vi "CTRE_PigeonIMU_UpdateUsage.vi"(10 "Usage":T1 items=["Defaul"=0, "ConnectCAN"=1, "ConnectTalonSRX"=2, "GetCompass"=134217728, "GetYPR"=268435456, "GetFused"=536870912, "GetAccel"=1073741824, "TempComp"=2147483648], 11 "PigeonIMUDevRef":T2={"DeviceStatus"={"status"=FALSE, "code"=0, "source"=""}, "Device Number"=0, "Type"=352321536, "Device ID"=0} {"Type" items=["CAN"=352321536, "TalonSRX"=33554432]}) -> ()   [LabVIEW 2016]
uses:
  <vilib>/Rock Robotics/WPI/ThirdParty/Sensors/Pigeon IMU/CTRE_PigeonIMU_DeviceRef.ctl
  <vilib>/Rock Robotics/WPI/ThirdParty/Sensors/Pigeon IMU/CTRE_PigeonIMU_ConnectionType.ctl
  <vilib>/Rock Robotics/WPI/ThirdParty/Sensors/Pigeon IMU/CTRE_PigeonIMU_UsageTypes.ctl
  <vilib>/Rock Robotics/WPI/ThirdParty/Sensors/Pigeon IMU/CTRE_PigeonIMU_GlobalOps.ctl
  <vilib>/Rock Robotics/WPI/ThirdParty/CanMotor/TalonSRX/WPI_CANTalonSRX_GlobalOps.ctl
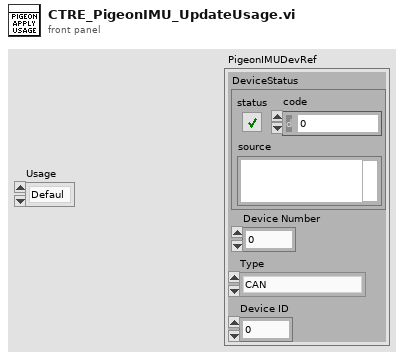
[diagram p1: front panel]
types:
  T1 = typedef "CTRE_PigeonIMU_UsageTypes.ctl" = u32
  T2 = typedef "CTRE_PigeonIMU_DeviceRef.ctl" = cluster{"DeviceStatus":errorcluster, "Device Number":u8, "Type":T3, "Device ID":u32}
  T3 = typedef "CTRE_PigeonIMU_ConnectionType.ctl" = u32
  T4 = typedef "CTRE_PigeonIMU_GlobalOps.ctl" = enum16{"Read For Send", "Write Error", "Get All", "Set Control Frame Rate", "Set Enable Frame Rate", "Write After Receive Fused Heading", "Write After Receive YPR", "Write After Receive Status", "Write After Receive Raw Magnetomoter", "Write After Receive Biased Magnetometer", "Write After Receive Biased Accelerometer", "Write After Receive Gyro", "Write After Receive Acceleromter Angles", "Write After Receive Startup Status", "Write After Receive Compass", "Write After Receive Quaternian", "Write After Receive AccumGyro", "Set Usage Frame"}
  T5 = typedef "CTRE_PigeonIMU_GlobalStatus.ctl" = cluster{"PigeonState":T6, "FusedHeading":cluster{"Heading":dbl, "Valid?":bool, "Fusing?":bool}, "YPR":cluster{"Yaw":dbl, "Pitch":dbl, "Roll":dbl}, "Compass":cluster{"Heading":dbl, "Magnitude":dbl, "Absolute Heading":dbl}, "Accelerometer":cluster{"Biased":cluster{"X":i16, "Y":i16, "Z":i16, "Norm":i16}, "Angles":cluster{"XZ Tilt":dbl, "YZ Tilt":dbl, "XY Tilt":dbl}}, "Magnetometer":cluster{"Raw":cluster{"X":i16, "Y":i16, "Z":i16}, "Biased":cluster{"X":i16, "Y":i16, "Z":i16}}, "Gyro":cluster{"X":dbl, "Y":dbl, "Z":dbl, "Norm":dbl}, "6D Quaternian":cluster{"W":dbl, "X":dbl, "Y":dbl, "Z":dbl}, "Temp. (C)":dbl, "UpTime":u32, "StartupStatus":cluster{"ResetCount":i32, "ResetFlags":i32, "FirmwareVersion":i32, "HasReset?":bool}, "Calibration":cluster{"CurrentMode":T7, "LastCalError":i32, "CalBooting?":bool}, "CAN Error":errorcluster, "AccumGyro":cluster{"X":dbl, "Y":dbl, "Z":dbl}, "Usage Frame":u32}
  T6 = typedef "CTRE_PigeonIMU_PigeonState.ctl" = enum16{"NoComm", "Initializing", "Ready", "UserCalibration"}
  T7 = typedef "CTRE_PigeonIMU_CalibrationMode.ctl" = u16
  T8 = typedef "WPI_CANTalonSRX_GlobalOps.ctl" = enum16{"Read For Send", "Write After Receive General", "Write After Receive Feedback", "Write After Receive Encoder", "Write After Receive Ain", "Write Error", "Get All", "Set Output", "Set Mode", "Set Master ID", "Set Brake Mode", "Set Reverse Feedback Sensor", "Set Reverse Closed Loop Output", "Set Override Limits", "Set Forward Limit Enabled", "Set Reverse Limit Enabled", "Set Feedback Select", "Set Profile Select", "Set Throttle Ramp Rate", "Disable", "Set Enc Codes Per Rev", "Set Num Pot Turns", "Set Control Frame Rate", "Enable Legacy Control", "Write After Receive Pulse Width", "Set Enable Frame Rate", "Write After Receive Motion Profile", "Set Motion Profile Flow Control", "Set Motion Profile Control Frame Rate", "Set Current Limit Enable", "Set Usage Frame"}
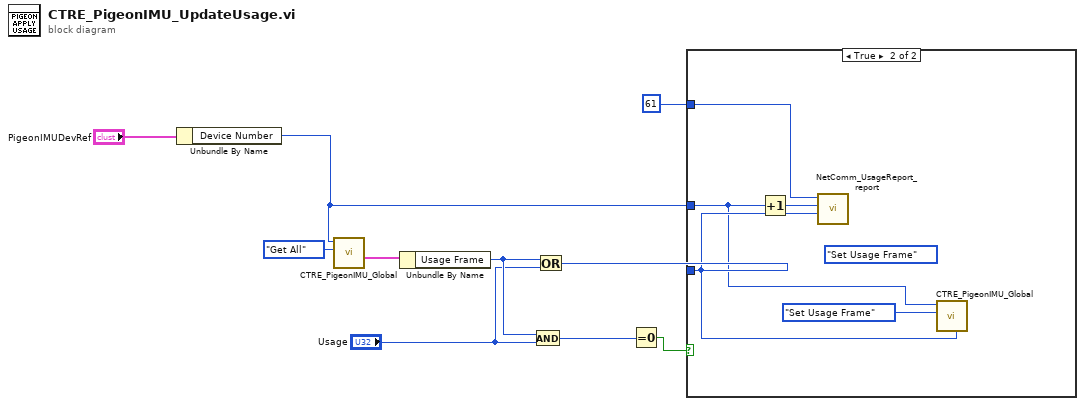
[diagram p0: block diagram]
diagram:
  n1 = Unbundle By Name("PigeonIMUDevRef") -> ("Device Number"=w2:u8)
  n2 = call <vilib>:"CTRE_PigeonIMU_Global.vi"("Operation"=CTRE_PigeonIMU_GlobalOps."Get All", "Device ID (0)"=w2) -> ("Get All"=w4:T5)  [unwired: 7 in, 2 out]
  n3 = Unbundle By Name(w4) -> ("Usage Frame"=w3:u32)
  n4 = And(x=w3, y="Usage") -> (x .and. y?=w9:T1)
  n5 = Or(x=w3, y="Usage") -> (x .or. y?=w8:T1)
  n6 = Equal To 0?(x=w9) -> (x = 0?=w10:bool)
  n7 = case shown="True" w10 {
    tunnel: 61 -> [_ w15]
    tunnel: w2 -> [_ w11]
    tunnel: w8 -> [_ w12]
    frame False {
    }
    frame True {
      (unwired) WPI_CANTalonSRX_GlobalOps."Set Usage Frame" ("Operation")
      n8 = Increment(x=w11) -> (x+1=w14:u8)
      n9 = call <vilib>:"NetComm_UsageReport_report.vi"("Context"=w12, "Instance Number"=w14, "Resource Type"=w15) -> ()  [unwired: 9 in]
      n10 = call <vilib>:"CTRE_PigeonIMU_Global.vi"("32-bit Frame"=w12, "Operation"=CTRE_PigeonIMU_GlobalOps."Set Usage Frame", "Device ID (0)"=w11) -> ()  [unwired: 6 in, 3 out]
    }
  }
